vi "BuzzXXI Main.vi"() -> ()   [LabVIEW 2015]
uses:
  Typedefs/GamepadData.ctl
  Typedefs/ActuatorInputs.ctl
  Typedefs/SensorInputData.ctl
  Typedefs/HMI_to_Control.ctl
  Typedefs/Shooter States.ctl
  Typedefs/CollectorLiftStates.ctl
  Typedefs/Hood States.ctl
  <vilib>/Platform/TimedLoop/XDataNode/timing_clust.ctl
  <vilib>/Platform/TimedLoop/XDataNode/nitl_modes.ctl
  <vilib>/Platform/TimedLoop/XDataNode/wakeup.ctl
  Typedefs/JoysticksGlobal.vi
  Gensubs/Bert_or_Ernie.vi
  Peripherals/Buzz XXI Peripherals/Nav X Library/NavX Global Data.vi
  <vilib>/Platform/TimedLoop/XDataNode/XDataNode.xnode
  <vilib>/Platform/TimedLoop/XDataNode/XDNodeRunTimeDep.lvlib
  <vilib>/NI_Real-Time Target Support.lvlib
  Peripherals/Buzz XXI Peripherals/Nav X Library/navX-MXP Library/navX-MXP IMU.lvlib
panel:
  out "Nav X Opened?":bool
  out "Error":errorcluster
  in  "On Comp":bool=TRUE
  out "HMI to ControlOut":T1={"RightDriveValue"=0.0, "LeftDriveValue"=0.0, "Intake Value"=0.0, "Shooter States"=enum."Shooter Off", "Collector Lift States"=enum."Collector Manual", "Shooter Hood States"=enum."Hood Close Shot", "Fire "=FALSE, "Collector Lift Manual Value"=0.0, "Shooter Hood Manual Value"=0.0, " Autolift portcullis"=FALSE, "Autoadjust CDF"=FALSE, "Hood Manual Request"=FALSE, "Collect Lift Manual Request"=FALSE, "Keep at target "=FALSE, "Hood Manual No."=0, "Collect Lift Manual No. "=0}
  in  "HMI to Control":T1={"RightDriveValue"=0.0, "LeftDriveValue"=0.0, "Intake Value"=0.0, "Shooter States"=enum."Shooter Off", "Collector Lift States"=enum."Collector Manual", "Shooter Hood States"=enum."Hood Close Shot", "Fire "=FALSE, "Collector Lift Manual Value"=0.0, "Shooter Hood Manual Value"=0.0, " Autolift portcullis"=FALSE, "Autoadjust CDF"=FALSE, "Hood Manual Request"=FALSE, "Collect Lift Manual Request"=FALSE, "Keep at target "=FALSE, "Hood Manual No."=0, "Collect Lift Manual No. "=0}
  out "SensorInputDataOut":T5
  in  "SensorInputData":T5
  in  "ActuatorInputs":T6
  in  "GamepadData":T7
  out "ActuatorInputsOut":T6
  out "GamepadDataOut":T7
  out "Finished Late? [i-1]":bool
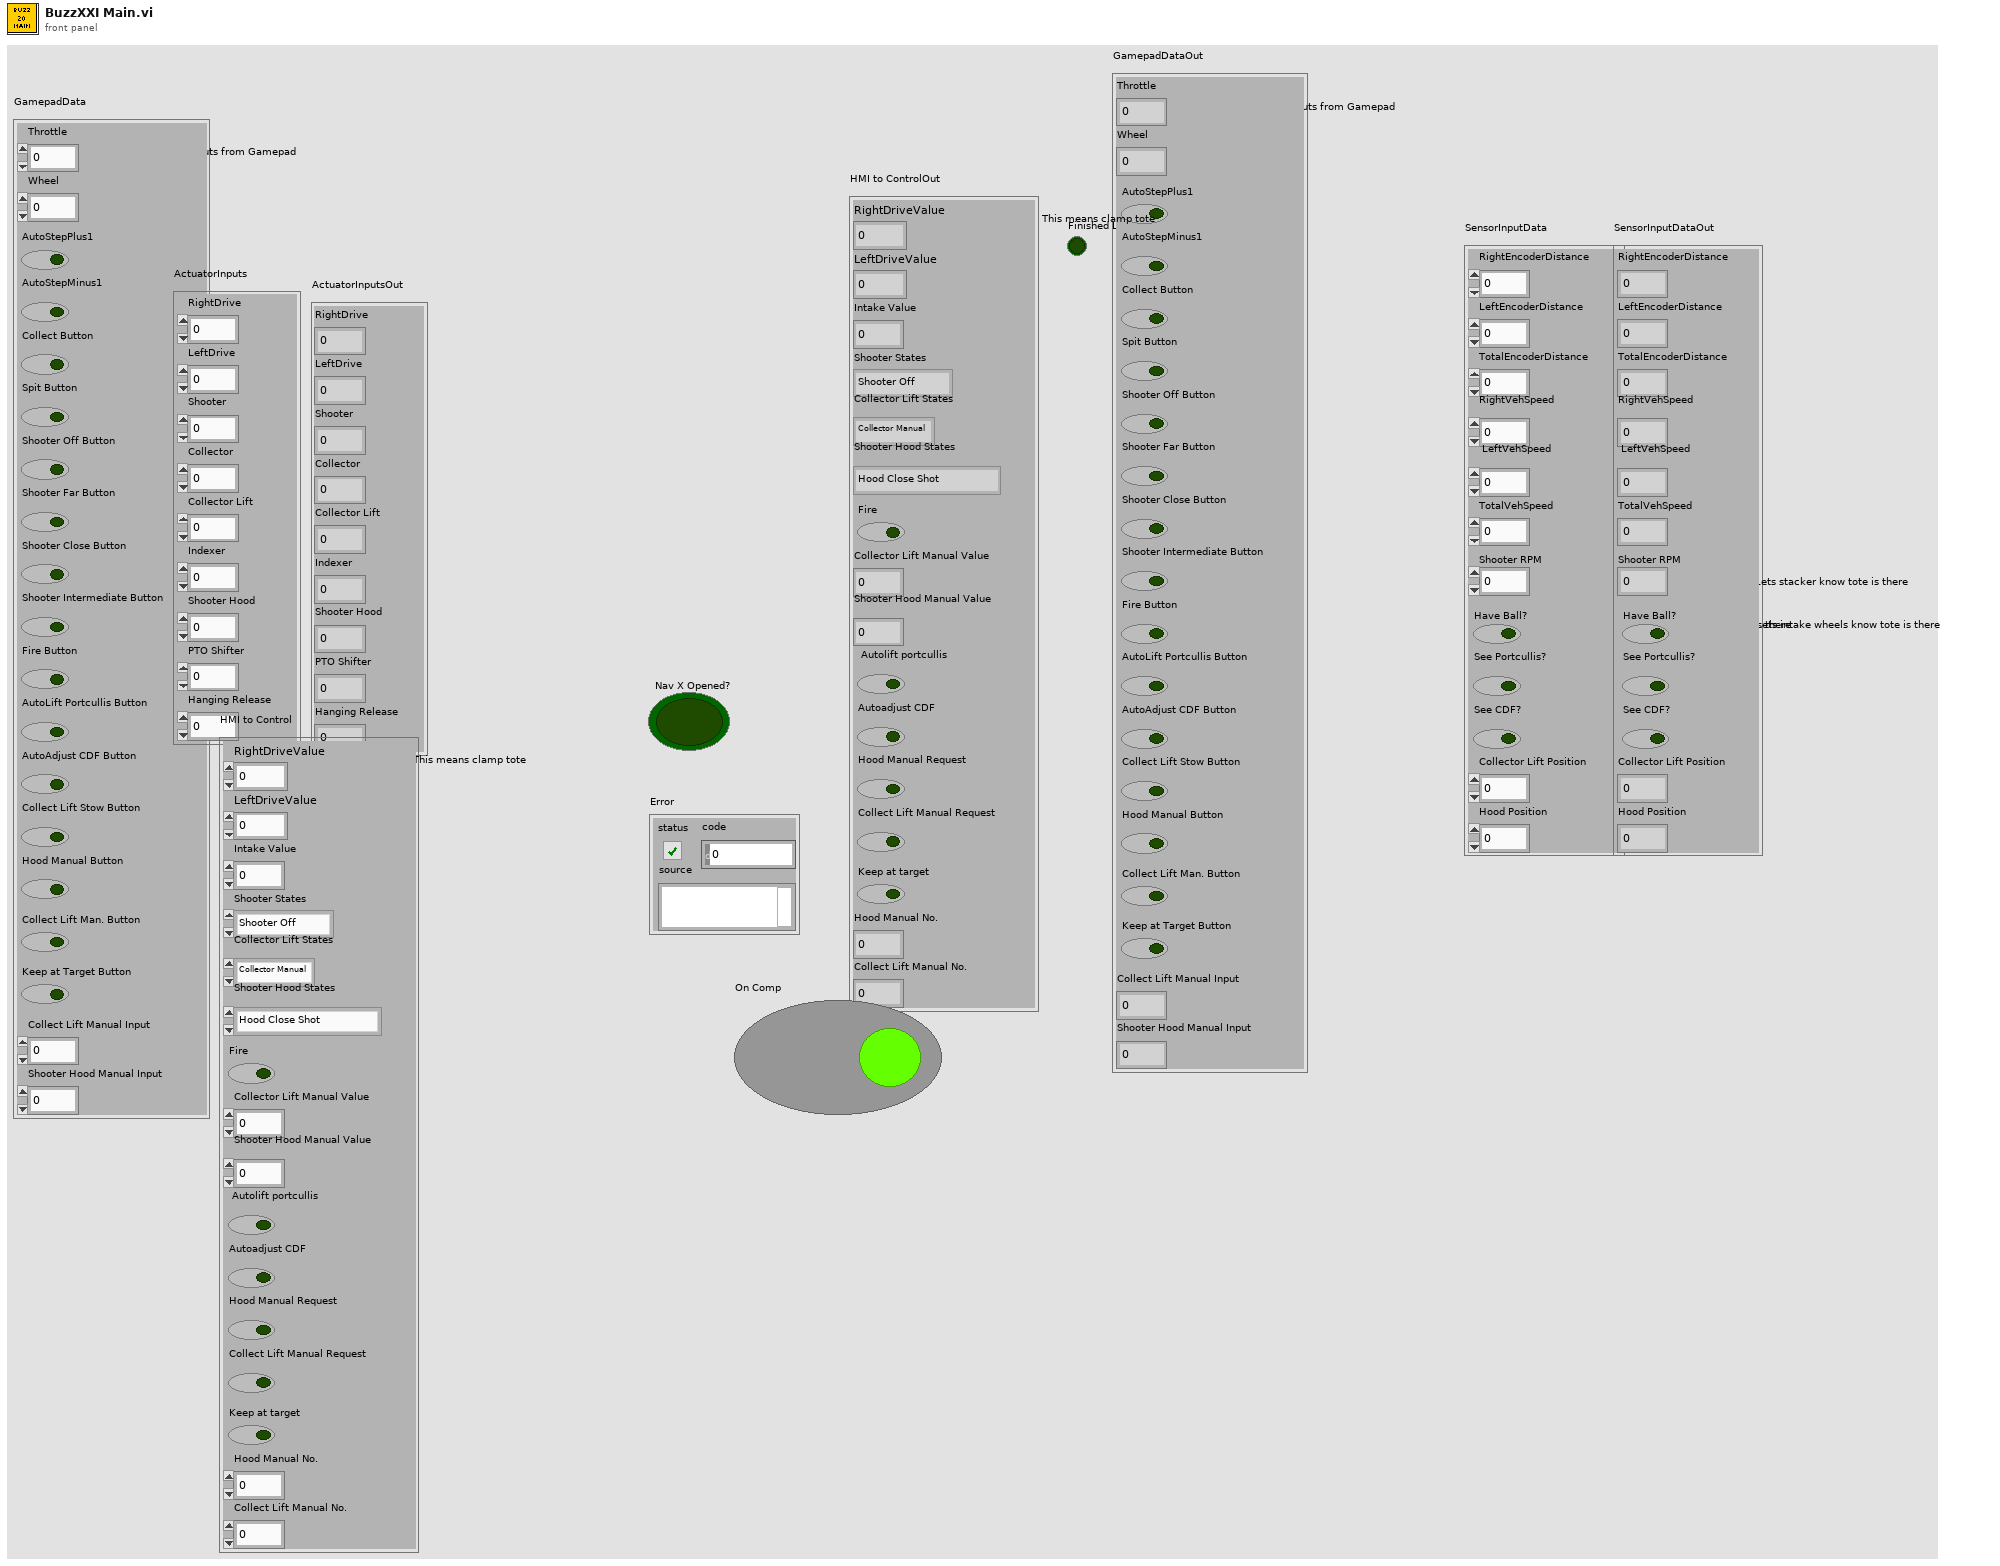
[diagram p1: front panel]
types:
  T1 = typedef "HMI_to_Control.ctl" = cluster{"RightDriveValue":dbl, "LeftDriveValue":dbl, "Intake Value":dbl, "Shooter States":T2, "Collector Lift States":T3, "Shooter Hood States":T4, "Fire ":bool, "Collector Lift Manual Value":dbl, "Shooter Hood Manual Value":dbl, " Autolift portcullis":bool, "Autoadjust CDF":bool, "Hood Manual Request":bool, "Collect Lift Manual Request":bool, "Keep at target ":bool, "Hood Manual No.":i8, "Collect Lift Manual No. ":i8}
  T2 = typedef "Shooter States.ctl" = enum16{"Shooter Off", "Shooter Far", "Shooter Close", "Shooter Intermediate", "Shooter Spy"}
  T3 = typedef "CollectorLiftStates.ctl" = enum16{"Collector Manual", "Stow", "Collect Position", "Spit Position", "Portcullis Set Up", "Portcullis Lift Up", "CDF Set Up", "Push CDF Down"}
  T4 = typedef "Hood States.ctl" = enum16{"Hood Manual ", "Hood Close Shot", "Hood Far Shot", "Hood Spy Shot", "Hood Intermediate"}
  T5 = typedef "SensorInputData.ctl" = cluster{"RightEncoderDistance":dbl, "LeftEncoderDistance":dbl, "TotalEncoderDistance":dbl, "RightVehSpeed":dbl, "LeftVehSpeed":dbl, "TotalVehSpeed":dbl, "Shooter RPM":dbl, "Have Ball?":bool, "See Portcullis?":bool, "See CDF?":bool, "Collector Lift Position":dbl, "Hood Position":dbl}
  T6 = typedef "ActuatorInputs.ctl" = cluster{"RightDrive":dbl, "LeftDrive":dbl, "Shooter":dbl, "Collector":dbl, "Collector Lift":dbl, "Indexer":dbl, "Shooter Hood":dbl, "PTO Shifter":dbl, "Hanging Release":dbl}
  T7 = typedef "GamepadData.ctl" = cluster{"Throttle":dbl, "Wheel":dbl, "AutoStepPlus1":bool, "AutoStepMinus1":bool, "Collect Button":bool, "Spit Button":bool, "Shooter Off Button":bool, "Shooter Far Button":bool, "Shooter Close Button":bool, "Shooter Intermediate Button":bool, "Fire Button":bool, "AutoLift Portcullis Button":bool, "AutoAdjust CDF Button":bool, "Collect Lift Stow Button":bool, "Hood Manual Button":bool, "Collect Lift Man. Button":bool, "Keep at Target Button":bool, "Collect Lift Manual Input":dbl, "Shooter Hood Manual Input":dbl}
  T8 = typedef "WPI_EncoderDevRef.ctl" = cluster{"DevStatus":errorcluster, "EncoderIndex":T9, "CounterIndex":T10, "DistancePerCount":dbl, "Decoding Type":T11}
  T9 = typedef "FPGA_EncoderIdx.ctl" = enum8{"Enc 0", "Enc 1", "Enc 2", "Enc 3", "Enc 4", "Enc 5", "Enc 6", "Enc 7", "Invalid"}
  T10 = typedef "FPGA_CounterCtrSystemIndex.ctl" = enum8{"Ctr 0", "Ctr 1", "Ctr 2", "Ctr 3", "Ctr 4", "Ctr 5", "Ctr 6", "Ctr 7", "Invalid"}
  T11 = typedef "WPI_EncoderType.ctl" = enum16{"1x", "2x", "4x"}
  T12 = typedef "WPI_CounterDevRef.ctl" = cluster{"DevStatus":errorcluster, "CntIndex":T10}
  T13 = typedef "WPI_SwitchDevRef.ctl" = cluster{"DevStatus":errorcluster, "DIO Channel":T14, "CntIndex":T10, "Normally Closed":bool}
  T14 = typedef "FPGA_DIOChannel.ctl" = enum8{"DIO 0", "DIO 1", "DIO 2", "DIO 3", "DIO 4", "DIO 5", "DIO 6", "DIO 7", "DIO 8", "DIO 9", "DIO MXP 0", "DIO MXP 1", "DIO MXP 2", "DIO MXP 3", "DIO MXP 4", "DIO MXP 5", "DIO MXP 6", "DIO MXP 7", "DIO MXP 8", "DIO MXP 9", "DIO MXP 10", "DIO MXP 11", "DIO MXP 12", "DIO MXP 13", "DIO MXP 14", "DIO MXP 15", "Invalid"}
  T15 = typedef "WPI_PotentiometerDevRef.ctl" = cluster{"DevStatus":errorcluster, "Analog Channel":T16, "Invert Output":bool}
  T16 = typedef "FPGA_AIChannel.ctl" = enum8{"AI 0", "AI 1", "AI 2", "AI 3", "AI MXP 0", "AI MXP 1", "AI MXP 2", "AI MXP 3", "Invalid"}
  T17 = typedef "WPI_MotorControlDeviceRef.ctl" = cluster{"DeviceStatus":errorcluster, "Type":T18, "PWM":cluster{"PWM Channel":T19, "DeadBand":T20}, "CAN":cluster{"Device Number":u8, "Control Mode":T21, "Semaphore":T22, "Max Vout":dbl, "TalonSRX Control Mode":T23}, "Invert":bool}
  T18 = typedef "WPI_MotorControlType.ctl" = enum16{"PWM", "CAN", "CANTalonSRX"}
  T19 = typedef "FPGA_DIOPWMChannel.ctl" = enum8{"PWM 0", "PWM 1", "PWM 2", "PWM 3", "PWM 4", "PWM 5", "PWM 6", "PWM 7", "PWM 8", "PWM 9", "PWM MXP 0", "PWM MXP 1", "PWM MXP 2", "PWM MXP 3", "PWM MXP 4", "PWM MXP 5", "PWM MXP 6", "PWM MXP 7", "PWM MXP 8", "PWM MXP 9", "Invalid"}
  T20 = typedef "WPI_PWMDeadband.ctl" = cluster{"Name":string, "maxPositivePwm":i32, "minPositivePwm":i32, "centerPwm":i32, "maxNegativePwm":i32, "minNegativePwm":i32, "angularRange":u16}
  T21 = typedef "WPI_CANJaguar_ControlMode.ctl" = enum8{"Percent VBus", "Current", "Speed", "Position", "Voltage"}
  T22 = typedef "Semaphore RefNum" = refnum<k1>
  T23 = typedef "WPI_CANTalonSRX_APIControlMode.ctl" = enum8{"Percent VBus", "Speed", "Position", "Slave", "Unchanged / Invalid", "Voltage Compensation", "Current", "Motion Profile"}
  T24 = typedef "WPI_ServoDeviceRef.ctl" = cluster{"DeviceStatus":errorcluster, "PWM Channel":T19, "DeadBand":T20}
  T25 = typedef "WPI_JoystickDevRef.ctl" = cluster{"Device":T26}
  T26 = typedef "WPI_JoystickDeviceEnum.ctl" = enum16{"USB 0", "USB 1", "USB 2", "USB 3", "USB 4", "USB 5"}
  T27 = typedef "navX-MXP IMU.lvlib/navX Device TypeDef.ctl" = cluster{"navX Interface Protocol":T28, "navX Interface Protocol TypeDefs":cluster{"SPIDevRef":T29, "I2CDevRef":T31}, "navX System Information":cluster{"Board Information":T33, "Status":T34, "Offsets":T38}, "navX Common Information":cluster{"Update Rate (4Hz-60Hz)":T39, "refnum name":string, "error":errorcluster}}
  T28 = typedef "navX-MXP IMU.lvlib/navX Interface Protocol.ctl" = enum16{"SPI", "I2C"}
  T29 = typedef "WPI_SPIDevRef.ctl" = cluster{"DevStatus":errorcluster, "Handle":i32, "SPI Bus":T30}
  T30 = typedef "spi_bus.ctl" = enum16{"SPI On-Board, CS0", "SPI On-Board, CS1", "SPI On-Board, CS2", "SPI On-Board, CS3", "SPI MXP", "Invalid"}
  T31 = typedef "WPI_I2CDevRef.ctl" = cluster{"DevStatus":errorcluster, "Device Address":u8, "Handle":i32, "I2C Bus":T32}
  T32 = typedef "i2c_bus.ctl" = enum16{"I2C On-Board", "I2C MXP", "Invalid"}
  T33 = typedef "navX-MXP IMU.lvlib/navX Board Information.ctl" = cluster{"WhoAmI (50 | 0x32)":u8, "Board Revision":u8, "Firmware Major Version":u8, "Firmware Minor Version":u8}
  T34 = typedef "navX-MXP IMU.lvlib/navX Status Data.ctl" = cluster{"Update Rate Hz":u8, "Accelerometer Full-Scale Range":u8, "Gyro Full-Scale Range":u16, "NAVX_OP_STATUS":T35, "NAVX_CAL_STATUS":T36, "NAVX_SELFTEST_STATUS":u8, "NAVX_SENSOR_STATUS":T37}
  T35 = typedef "navX-MXP IMU.lvlib/navX NAVX_OP_STATUS.ctl" = u8
  T36 = typedef "navX-MXP IMU.lvlib/navX NAVX_CAL_STATUS.ctl" = u8
  T37 = typedef "navX-MXP IMU.lvlib/navX NAVX_SENSOR_STATUS.ctl" = cluster{"MOVING":bool, "YAW_STABLE":bool, "MAG_DISTURBANCE":bool, "ALTITUDE_VALID":bool, "SEALEVEL_PRESS_SET":bool, "FUSED_HEADING_VALID":bool}
  T38 = typedef "navX-MXP IMU.lvlib/navX Offsets Data.ctl" = cluster{"Yaw":dbl, "Quat W":dbl, "Quat X":dbl, "Quat Y":dbl, "Quat Z":dbl}
  T39 = typedef "navX-MXP IMU.lvlib/navX Update Rate.ctl" = u8
  T40 = typedef "XDNodeRunTimeDep.lvlib/timing_clust.ctl" = cluster{"Expected End [f-1]":u64, "Actual End [f-1]":u64, "Finished Late? [f-1]":bool, "Expected End [i-1]":u64, "Actual End [i-1]":u64, "Finished Late? [i-1]":bool, "Expected Start [i]":u64, "Actual Start [i]":u64, "Expected Start [f]":u64, "Actual Start [f]":u64, "Source Name":string, "Structure Name":string, "Period":i64, "Deadline":i64, "Offset":i64, "Start":i64, "Priority":i32, "Timeout":i32, "Mode":T41, "Wakeup Reason":T42, "Error":errorcluster, "Source Type":string, "Secondary Source Type":string, "Global End Time":u64, "Global Start Time":u64, "Frame Duration":u64, "Iteration Duration":u64, "Assigned CPU":i32, "I/O Scan Engine Mode":u32}
  T41 = typedef "XDNodeRunTimeDep.lvlib/nitl_modes.ctl" = enum32{"No Change", "Process missed periods, maintain original phase", "Discard missed periods, maintain original phase", "Process missed periods, ignore original phase", "Discard missed periods, ignore original phase"}
  T42 = typedef "XDNodeRunTimeDep.lvlib/wakeup.ctl" = enum32{"Normal", "Aborted", "Asynchronous wakeup", "Timing source error", "Timed loop error", "Timeout"}
  T43 = typedef "navX-MXP IMU.lvlib/navX YPRH Data.ctl" = cluster{"Yaw":dbl, "Pitch":dbl, "Roll":dbl, "Heading":dbl}
  T44 = typedef "NetComm_ControlWord.ctl" = cluster{"Enabled":bool, "Autonomous":bool, "Test":bool, "E-Stop":bool, "FMS Attached":bool, "DS Attached":bool}
  T45 = typedef "WPI_DriverStationRobotMode2.ctl" = enum16{"Autonomous Disabled", "Autonomous Enabled", "Teleop Disabled", "Teleop Enabled", "Disconnected", "Finish", "Test Disabled", "Test Enabled", "Emergency Stopped"}
  T46 = cluster{"Axes":dbl[], "Buttons":bool[], "POVs":i16[]}
  T47 = cluster{cluster{"Axes":dbl[], "Buttons":bool[], "POVs":i16[]}, cluster{"Axes":dbl[], "Buttons":bool[], "POVs":i16[]}}
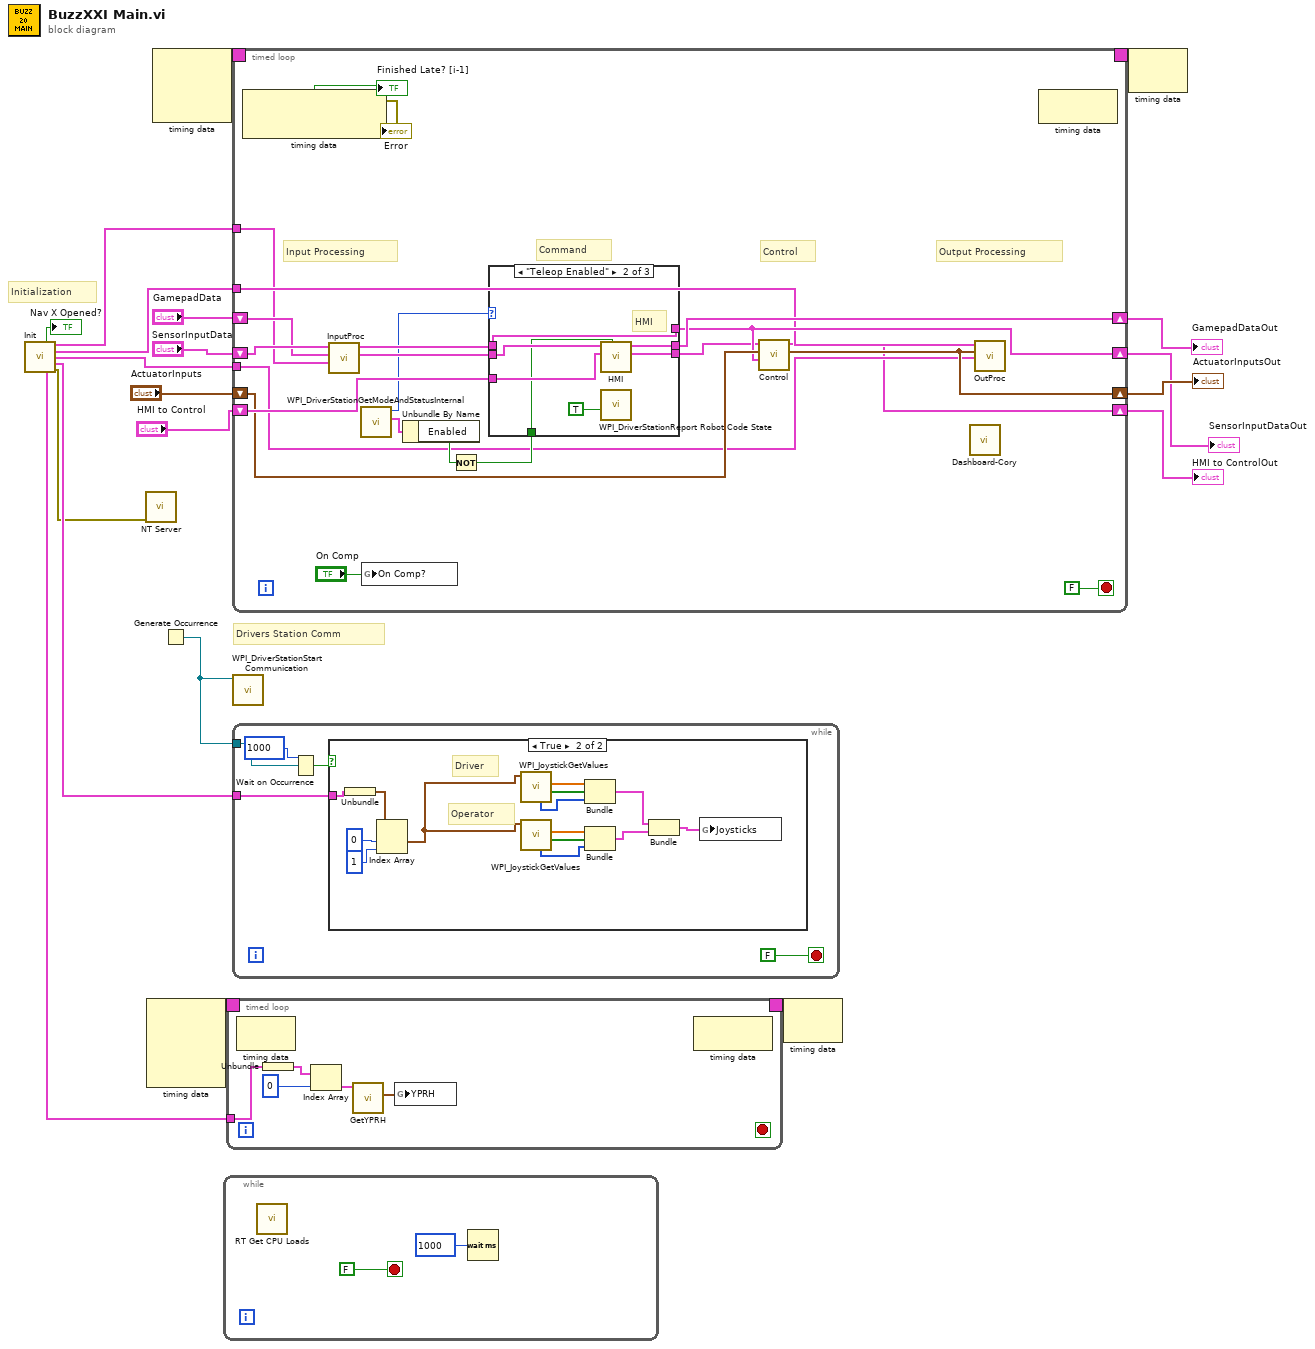
[diagram p0: block diagram]
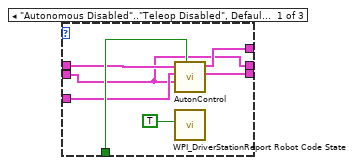
[diagram p3: hidden frame]
diagram:
  # "Drivers Station Comm"
  # "Initialization"
  n1 = call "Init.vi"() -> ("Nav X Opened?"=→"Nav X Opened?":bool, "Sensors"=w4:cluster{T8[], T12[], T13[], T15[]}, "Motors"=w3:cluster{T17[]}, "Servos"=w2:cluster{T24[]}, "Joysticks"=w6:cluster{T25[]}, "NavX"=w7:cluster{T27[]}, "Nav X Error"=w1:errorcluster)  [unwired: 9 in]
  n2 = call <vilib>:"NT Server.vi"("error in (no error)"=w1) -> ()  [unwired: 11 in]
  n3 = node-c288() -> (w9:T40)  [unwired: 4 in]
  n4 = node-c288() -> (w20:T40)  [unwired: 3 in]
  n5 = Generate Occurrence() -> (w10:refnum<k4>)
  n6 = while {
    stop <- FALSE stop-if-true
    n7 = call <vilib>:"RT Get CPU Loads.vi"() -> ()  [unwired: 10 in, 2 out]
    n8 = Wait (ms)(milliseconds to wait=u32 1000) -> ()  [unwired: 1 out]
  }
  n9 = timed-loop {
    timing: w9 -> [_]
    timing-out: [_] -> w8
    tunnel: w7 -> [w25]
    stop <- _ stop-if-true
    n10 = node-c288() -> ()  [unwired: 1 in, 1 out]
    n11 = Unbundle(w25) -> (w24:T27[])
    n12 = Index Array(array=w24, index=0) -> (element=w23:T27)
    n13 = call "GetYPRH.vi"("navX Device TypeDef"=w23) -> ("YPRH"=w26:T43)  [unwired: 8 in, 2 out]
    n14 = global write "NavX Global Data.vi" "YPRH"(w26) -> ()
    n15 = node-c288() -> ()  [unwired: 1 in, 1 out]
  }
  n16 = timed-loop {
    timing: w20 -> [_]
    timing-out: [_] -> w19
    shift-right: [w40] -> w18
    shift-left: "GamepadData" -> [w43]
    shift-right: [w38] -> w17
    shift-left: "ActuatorInputs" -> [w39]
    shift-right: [w30] -> w11
    shift-left: "HMI to Control" -> [w41]
    shift-right: [w36] -> w13
    shift-left: "SensorInputData" -> [w44]
    tunnel: w4 -> [w32]
    tunnel: w3 -> [w34]
    tunnel: w2 -> [w33]
    stop <- FALSE stop-if-true
    # "Output Processing"
    # "Control"
    # "Command"
    # "Input Processing"
    n17 = node-c288() -> (→"Finished Late? [i-1]":bool, →"Error":errorcluster)  [unwired: 1 in]
    n18 = call "InputProc.vi"("Sensors"=w32, "Gamepad Data"=w43, "SensorInputData"=w44) -> ("Gamepad Data Out"=w42:T7, "SensorInputDataOut"=w37:T5)  [unwired: 6 in]
    n19 = call <vilib>:"WPI_DriverStationGetModeAndStatusInternal.vi"() -> ("Control Word"=w47:T44, "Robot Mode"=w31:T45)  [unwired: 10 in]
    n20 = global write "Bert_or_Ernie.vi" "On Comp?"("On Comp") -> ()
    n21 = Unbundle By Name(w47) -> ("Enabled"=w46:bool)
    n22 = Not(x=w46) -> (.not. x?=w45:bool)
    n23 = case shown="\"Teleop Enabled\"" w31 {
      tunnel: w45 -> [w57 w59 _]
      tunnel: w42 -> [w52 w64 _]
      tunnel: w41 -> [w55 w63 _]
      tunnel: [w52 w62 _] -> w40
      tunnel: [w54 w61 _] -> w35
      tunnel: w37 -> [w56 w60 _]
      tunnel: [w53 w60 _] -> w36
      frame "Autonomous Disabled".."Teleop Disabled", Default {
        n24 = call "AutonControl.vi"("Disabled"=w57, "Gamepad Data"=w52, "HMI to Control"=w55, "SensorInputData"=w56) -> ("HMI to Control Out"=w54:T1, "SensorInputDataOut"=w53:T5)  [unwired: 5 in, 1 out]
        n25 = call <vilib>:"WPI_DriverStationReport Robot Code State.vi"("Autonomous"=TRUE) -> ()  [unwired: 10 in, 1 out]
      }
      frame "Teleop Enabled" {
        # "HMI"
        n26 = call "HMI.vi"("Disabled"=w59, "HMI to Control"=w63, "Gamepad Data"=w64) -> ("HMI to Control"=w61:T1, "Gamepad Data Out"=w62:T7)  [unwired: 5 in]
        n27 = call <vilib>:"WPI_DriverStationReport Robot Code State.vi"("TeleOp"=TRUE) -> ()  [unwired: 10 in, 1 out]
      }
      frame "Disconnected", "Emergency Stopped" {
      }
    }
    n28 = call "Control.vi"("SensorInputData"=w36, "ActuatorInputs"=w39, "HMI to Control"=w35) -> ("ActuatorInputs Out"=w38:T6, "HMI to Control Out"=w30:T1)  [unwired: 7 in]
    n29 = call "Dashboard-Cory.vi"() -> ()  [unwired: 10 in]
    n30 = call "OutProc.vi"("Servos"=w33, "ActuatorInputs"=w38, "Motors"=w34) -> ()  [unwired: 9 in]
    n31 = node-c288() -> ()  [unwired: 1 in, 1 out]
  }
  "GamepadDataOut" <- w18
  "ActuatorInputsOut" <- w17
  "SensorInputDataOut" <- w13
  "HMI to ControlOut" <- w11
  n32 = call <vilib>:"WPI_DriverStationStart Communication.vi"("occurrence"=w10) -> ()  [unwired: 1 in, 10 out]
  n33 = while {
    tunnel: w10 -> [w73]
    tunnel: w6 -> [w70]
    stop <- FALSE stop-if-true
    n34 = Wait on Occurrence(2:w73, 3:1000 ("ms timeout (-1)")) -> (0:w72:bool)  [unwired: 1 in]
    n35 = case shown="True" w72 {
      tunnel: w70 -> [_ w77]
      frame False {
      }
      frame True {
        # "Operator"
        # "Driver"
        n36 = Unbundle(w77) -> (w76:T25[])
        n37 = Index Array(array=w76, index #1=0 ("index"), index #2=1 ("index")) -> (element #1=w75:T25)  [unwired: 1 out]
        n38 = call <vilib>:"WPI_JoystickGetValues.vi"("JoystickDevRef"=w75) -> ("Buttons"=w85:bool[], "Axes"=w86:dbl[], "POVs"=w84:i16[])  [unwired: 6 in, 2 out]
        n39 = call <vilib>:"WPI_JoystickGetValues.vi"("JoystickDevRef"=w75) -> ("Buttons"=w82:bool[], "Axes"=w83:dbl[], "POVs"=w81:i16[])  [unwired: 6 in, 2 out]
        n40 = Bundle("Axes"=w86, "Buttons"=w85, "POVs"=w84) -> (w80:T46)  [unwired: 1 in]
        n41 = Bundle("Axes"=w83, "Buttons"=w82, "POVs"=w81) -> (w79:T46)  [unwired: 1 in]
        n42 = Bundle(w80, w79) -> (w78:T47)  [unwired: 1 in]
        n43 = global write "JoysticksGlobal.vi" "Joysticks"(w78) -> ()
      }
    }
  }
  n44 = node-c288(w8) -> ()  [unwired: 1 out]
  n45 = node-c288(w19) -> ()  [unwired: 1 out]
